vi "MaxEye_ATE_Create Configuration Value Header.vi"(9 "Class_value":string, 10 "Label_name":string, 11 "Class_name":string) -> (3 "Encoded Value":string)   [LabVIEW 2021]
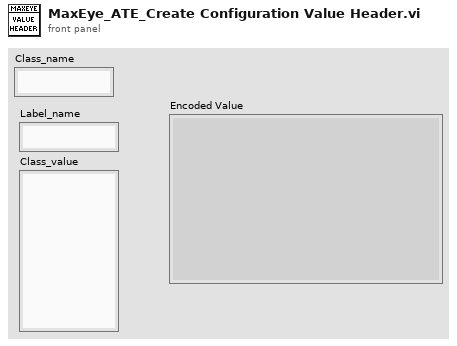
[diagram p1: front panel]
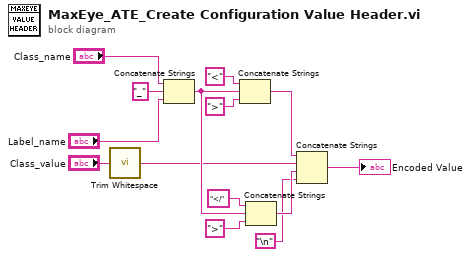
[diagram p0: block diagram]
diagram:
  n1 = call <vilib>:"Trim Whitespace.vi"("string"="Class_value") -> ("trimmed string"=w1:string)  [unwired: 1 in]
  n2 = Concatenate Strings("Class_name", "_" ("string"), "Label_name") -> (w3:string)
  n3 = Concatenate Strings("<" ("string"), w3, ">" ("string")) -> (w10:string)
  n4 = Concatenate Strings("</" ("string"), w3, ">" ("string")) -> (w9:string)
  n5 = Concatenate Strings(w10, w1, w9, "\n") -> (→"Encoded Value":string)
